vi "Barcode scanner UI.vi"() -> ()   [LabVIEW 2015]
uses:
  <vilib>/Utility/NIReport.llb/Append Report Text (str wrap).vi
  <vilib>/Utility/NIReport.llb/NI_report.lvclass
panel:
  out "STATUS":string
  out "MAC ID":string
  out "SERIAL NUMBER":string
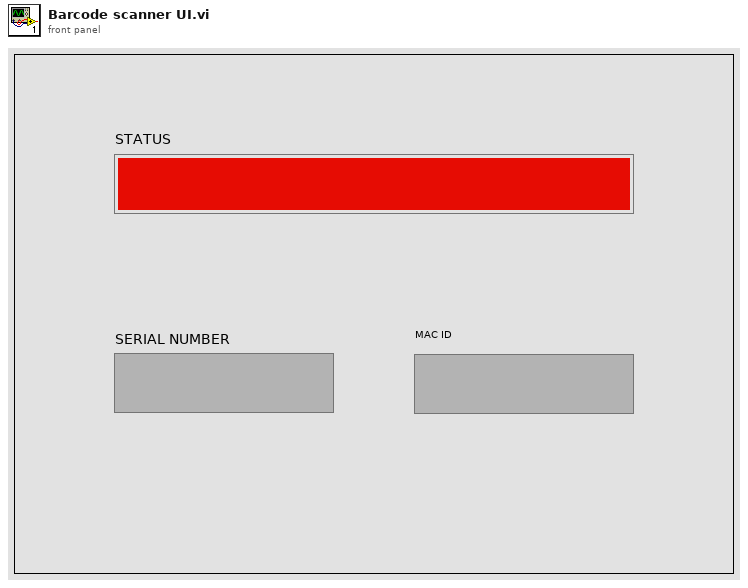
[diagram p1: front panel]
types:
  T1 = enum16{"Standard Report", "HTML", "Word", "Excel"}
  T2 = cluster{"Charset (-1)":i16, "Weight (-1)":i16, "Name":string, "Size":string}
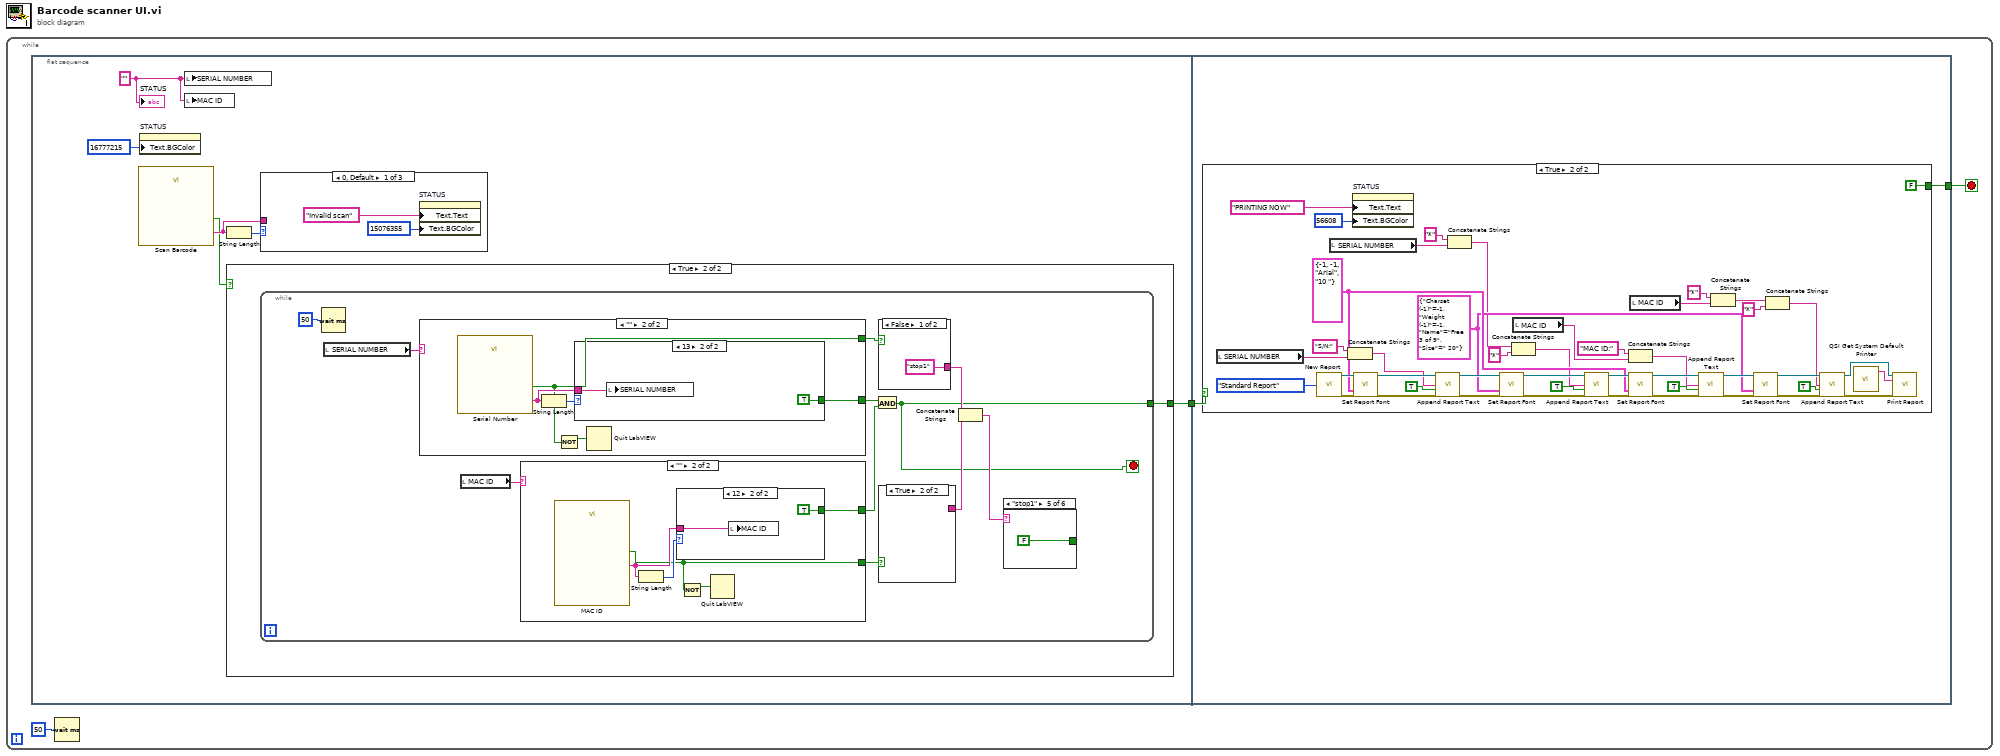
[diagram p0: block diagram]
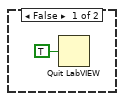
[diagram p2: hidden frame]
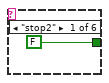
[diagram p3: hidden frame]
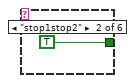
[diagram p4: hidden frame]
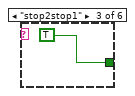
[diagram p5: hidden frame]
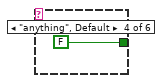
[diagram p6: hidden frame]
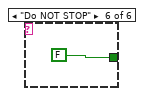
[diagram p7: hidden frame]
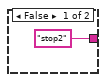
[diagram p9: hidden frame]
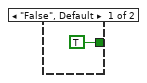
[diagram p10: hidden frame]
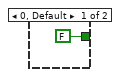
[diagram p11: hidden frame]
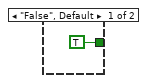
[diagram p12: hidden frame]
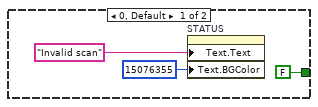
[diagram p13: hidden frame]
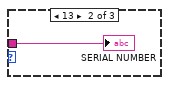
[diagram p14: hidden frame]
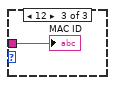
[diagram p15: hidden frame]
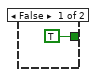
[diagram p16: hidden frame]
diagram:
  n1 = while {
    stop <- w2 stop-if-true
    n2 = flat-sequence {
      tunnel: [w4] -> w1
      tunnel: [w56] -> w2
      tunnel: w1 -> [w55]
      frame #0 {
        w6 = "" ("Serial Number")
        n3 = call "Scan Barcode"() -> ("Scan now"=w9:string, "Submit"=w5:bool)  [unwired: 17 in, 1 out]
        n4 = property on="STATUS" class="Str"("Text.BGColor"=u32 16777215 ("Text.Text Colors:BG Color")) -> ()  [unwired: 2 in, 2 out]
        n5 = local write "SERIAL NUMBER"(w6) -> ()
        n6 = local write "MAC ID"(w6) -> ()
        n7 = String Length(string=w9) -> (length=w8:i32)
        n8 = case shown="True" w5 {
          tunnel: [_ w11] -> w4
          frame False {
            n9 = Quit LabVIEW(quit? (T)=TRUE) -> ()
          }
          frame True {
            n10 = while {
              tunnel: [w12] -> w11
              stop <- w12 stop-if-true
              n11 = Wait (ms)(milliseconds to wait=u32 50) -> ()  [unwired: 1 out]
              n12 = local read "SERIAL NUMBER"() -> (w22:string)
              n13 = case shown="\"\"" w22 {
                tunnel: [TRUE w43] -> w19
                tunnel: [_ w41] -> w16
                frame "False", Default {
                }
                frame "" {
                  n14 = call "Serial Number"() -> ("Serial Number"=w44:string, "Submit"=w41:bool)  [unwired: 17 in, 1 out]
                  n15 = String Length(string=w44) -> (length=w45:i32)
                  n16 = Not(x=w41) -> (.not. x?=w42:bool)
                  n17 = case shown="13" w45 {
                    tunnel: w44 -> [_ w50]
                    tunnel: [FALSE TRUE] -> w43
                    frame 0, Default {
                      n18 = property on="STATUS" class="Str"("Text.Text"="Invalid scan", "Text.BGColor"=u32 15076355 ("Text.Text Colors:BG Color")) -> ()  [unwired: 2 in, 2 out]
                    }
                    frame 13 {
                      n19 = local write "SERIAL NUMBER"(w50) -> ()
                    }
                  }
                  n20 = Quit LabVIEW(quit? (T)=w42) -> ()
                }
              }
              n21 = local read "MAC ID"() -> (w21:string)
              n22 = case shown="\"\"" w21 {
                tunnel: [TRUE w34] -> w18
                tunnel: [_ w32] -> w17
                frame "False", Default {
                }
                frame "" {
                  n23 = call "MAC ID"() -> ("Mac ID"=w36:string, "Submit"=w32:bool)  [unwired: 17 in, 1 out]
                  n24 = String Length(string=w36) -> (length=w35:i32)
                  n25 = case shown="12" w35 {
                    tunnel: w36 -> [_ w39]
                    tunnel: [FALSE TRUE] -> w34
                    frame 0, Default {
                    }
                    frame 12 {
                      n26 = local write "MAC ID"(w39) -> ()
                    }
                  }
                  n27 = Not(x=w32) -> (.not. x?=w33:bool)
                  n28 = Quit LabVIEW(quit? (T)=w33) -> ()
                }
              }
              n29 = And(x=w19, y=w18) -> (x .and. y?=w12:bool)
              n30 = case shown="False" w16 {
                tunnel: ["stop1" _] -> w15
                frame False {
                }
                frame True {
                }
              }
              n31 = case shown="True" w17 {
                tunnel: ["stop2" _] -> w14
                frame False {
                }
                frame True {
                }
              }
              n32 = Concatenate Strings(w15, w14) -> (w13:string)
              n33 = case shown="\"stop1\"" w13 {
                tunnel: [FALSE TRUE TRUE FALSE FALSE FALSE] -> _
                frame "stop2" {
                }
                frame "stop1stop2" {
                }
                frame "stop2stop1" {
                }
                frame "anything", Default {
                }
                frame "stop1" {
                }
                frame "Do NOT STOP" {
                }
              }
            }
          }
        }
        n34 = case shown="0, Default" w8 {
          tunnel: w9 -> [_ w53 w54]
          frame 0, Default {
            n35 = property on="STATUS" class="Str"("Text.Text"="Invalid scan", "Text.BGColor"=u32 15076355 ("Text.Text Colors:BG Color")) -> ()  [unwired: 2 in, 2 out]
          }
          frame 13 {
            "SERIAL NUMBER" <- w53
          }
          frame 12 {
            "MAC ID" <- w54
          }
        }
        "STATUS" <- w6
      }
      frame #1 {
        n36 = case shown="True" w55 {
          tunnel: [TRUE FALSE] -> w56
          frame False {
          }
          frame True {
            w73 = T2 {"Charset (-1)"=-1, "Weight (-1)"=-1, "Name"="Free 3 of 9", "Size"=" 20"} ("font settings")
            w81 = T2 {"Charset (-1)"=-1, "Weight (-1)"=-1, "Name"="Arial", "Size"="10 "} ("font settings")
            n37 = local read "SERIAL NUMBER"() -> (w83:string)
            n38 = call <vilib>:"New Report.vi"("report type"=T1."Standard Report") -> ("report out"=w102:refnum<class "NI_report.lvclass">, "error out"=w101:errorcluster)  [unwired: 13 in]
            n39 = local read "SERIAL NUMBER"() -> (w70:string)
            n40 = Concatenate Strings("S/N:" ("string"), w83) -> (w90:string)
            n41 = property on="STATUS" class="Str"("Text.Text"="PRINTING NOW" ("STATUS"), "Text.BGColor"=u32 56608 ("Text.Text Colors:BG Color")) -> ()  [unwired: 2 in, 2 out]
            n42 = call-dynamic "Set Report Font.vi"("report in"=w102, "font settings"=w81, "error in (no error)"=w101) -> ("report out"=w100:refnum<class "NI_report.lvclass">, "error out"=w99:errorcluster)  [unwired: 10 in, 1 out]
            n43 = call-poly <vilib>:"Append Report Text.vi"("report in"=w100, "text"=w90, "append on new line? (F)"=TRUE, "error in (no error)"=w99) -> ("report out"=w96:refnum<class "NI_report.lvclass">, "error out"=w95:errorcluster)  [unwired: 8 in, 2 out]
            n44 = Concatenate Strings("*" ("string"), w70) -> (w69:string)
            n45 = call-dynamic "Set Report Font.vi"("report in"=w96, "font settings"=w73, "error in (no error)"=w95) -> ("report out"=w93:refnum<class "NI_report.lvclass">, "error out"=w92:errorcluster)  [unwired: 10 in, 1 out]
            n46 = Concatenate Strings(w69, "*" ("string")) -> (w67:string)
            n47 = local read "MAC ID"() -> (w62:string)
            n48 = call-poly <vilib>:"Append Report Text.vi"("report in"=w93, "text"=w67, "append on new line? (F)"=TRUE, "error in (no error)"=w92) -> ("report out"=w82:refnum<class "NI_report.lvclass">, "error out"=w84:errorcluster)  [unwired: 8 in, 2 out]
            n49 = Concatenate Strings("MAC ID:" ("string"), w62) -> (w72:string)
            n50 = call-dynamic "Set Report Font.vi"("report in"=w82, "font settings"=w81, "error in (no error)"=w84) -> ("report out"=w85:refnum<class "NI_report.lvclass">, "error out"=w87:errorcluster)  [unwired: 10 in, 1 out]
            n51 = local read "MAC ID"() -> (w64:string)
            n52 = call-poly <vilib>:"Append Report Text.vi"("report in"=w85, "text"=w72, "append on new line? (F)"=TRUE, "error in (no error)"=w87) -> ("report out"=w77:refnum<class "NI_report.lvclass">, "error out"=w78:errorcluster)  [unwired: 8 in, 2 out]
            n53 = Concatenate Strings("*" ("string"), w64) -> (w65:string)
            n54 = call-dynamic "Set Report Font.vi"("report in"=w77, "font settings"=w73, "error in (no error)"=w78) -> ("report out"=w76:refnum<class "NI_report.lvclass">, "error out"=w79:errorcluster)  [unwired: 10 in, 1 out]
            n55 = Concatenate Strings(w65, "*" ("string")) -> (w61:string)
            n56 = call-poly <vilib>:"Append Report Text.vi"("report in"=w76, "text"=w61, "append on new line? (F)"=TRUE, "error in (no error)"=w79) -> ("report out"=w75:refnum<class "NI_report.lvclass">, "error out"=w74:errorcluster)  [unwired: 8 in, 2 out]
            n57 = call "QSI Get System Default Printer.vi"() -> ("System Default Printer"=w98:string)  [unwired: 4 in, 1 out]
            n58 = call-dynamic "Print Report.vi"("report in"=w75, "printer name (default)"=w98, "error in (no error)"=w74) -> ()  [unwired: 11 in, 2 out]
          }
        }
      }
    }
    n59 = Wait (ms)(milliseconds to wait=u32 50) -> ()  [unwired: 1 out]
  }
